vi "SystemClose.vi"(8 "error in (no error)":errorcluster, 10 "Pound":refnum<class "Pound.lvclass">, 11 "Qbus":refnum<class "Qbus.lvclass">) -> (0 "error out":errorcluster)   [LabVIEW 2015, in "System.lvlib"]
uses:
  System.lvlib
  <vilib>/addons/Qbus/Qbus.lvclass
  <vilib>/NI/Software Watchdog/Pound/Pound.lvclass
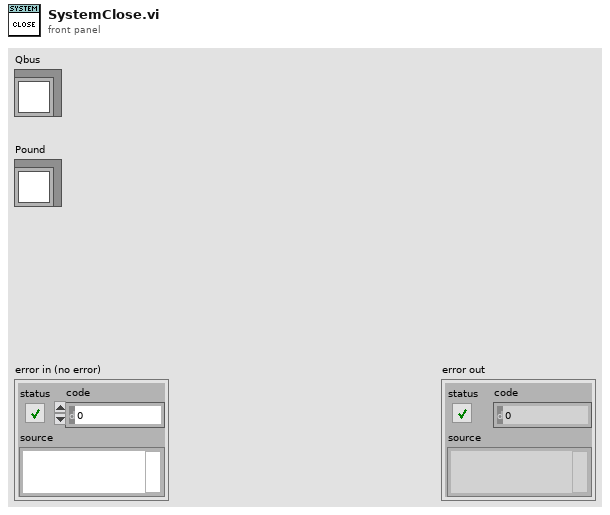
[diagram p1: front panel]
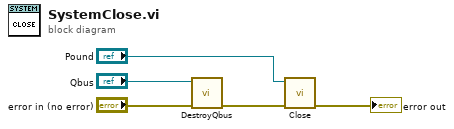
[diagram p0: block diagram]
diagram:
  n1 = call <vilib>:"DestroyQbus.vi"("error in (no error)"="error in (no error)", "Qbus"="Qbus") -> ("error in (no error)"=w4:errorcluster)  [unwired: 9 in]
  n2 = call <vilib>:"Close.vi"("error in (no error)"=w4, "Pound"="Pound") -> ("error out"=→"error out":errorcluster)  [unwired: 9 in]
